vi "Day 22-Add New.vi"(10 "Instruction in":cluster{i64[], i64}, 11 "Map in":map{i64[], i64}(c390)) -> (3 "Map out":map{i64[], i64}(c390))   [LabVIEW 2021]
uses:
  <vilib>/Utility/miscctls.llb/LVMapReplaceAction.ctl
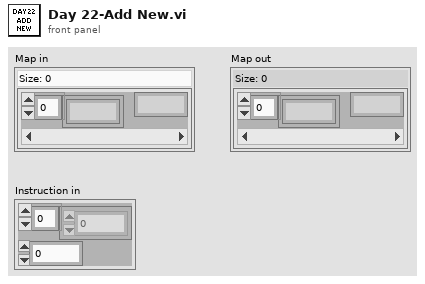
[diagram p1: front panel]
types:
  T1 = typedef "LVMapReplaceAction.ctl" = enum32{"Modify Entry only if found", "Add or Modify Entry", "Delete Entry"}
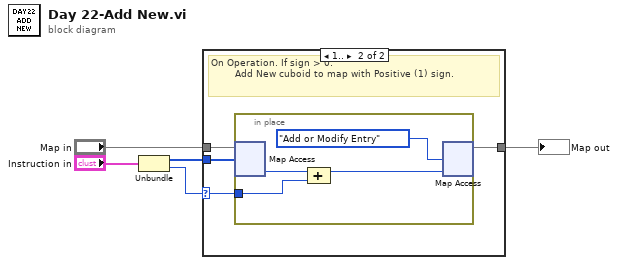
[diagram p0: block diagram]
diagram:
  n1 = Unbundle("Instruction in") -> (w4:i64[], w5:i64)
  n2 = case shown="1.." w5 {
    selector: w5 -> [_ w7]
    tunnel: w4 -> [_ w10]
    tunnel: "Map in" -> [w6 w9]
    tunnel: [w6 w8] -> w2
    frame Default {
      # "Off Operation"
    }
    frame 1.. {
      # "On Operation. If sign > 0:\n        Add New cuboid to map with Positive (1) sign."
      n3 = in-place {
        in-place-border: w7 -> [w11]
        n4 = in-place-map #1(w9, w10) -> (w13:i64)  [unwired: 1 in, 1 out]
        n5 = Compound Arithmetic op=ADD(w13, w11) -> (w12:i64)
        n6 = in-place-map #1(w12, LVMapReplaceAction."Add or Modify Entry" ("action")) -> (w8:map{i64[], i64})  [unwired: 2 out]
      }
    }
  }
  "Map out" <- w2
